vi "Periodic Tasks.vi"(8 "error in":errorcluster) -> ()   [LabVIEW 2017]
doc: "This VI runs in parallel to other tasks. It can contain as many user-defined periodic loops as you need. These can carry out PID or other sorts of timed response."
uses:
  Globals/Global_STOP.vi
  Systems/VisionHW Folder/VisionHW.lvlib
  Systems/Gimbal/Gimbal.lvlib
  _SHARE ALL/RoboRio Share All/Systems Share All/Joystick/Joystick.lvlib
panel:
  in  "Camera Occurance":refnum<k4>
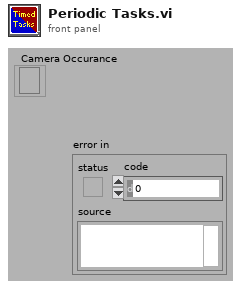
[diagram p1: front panel]
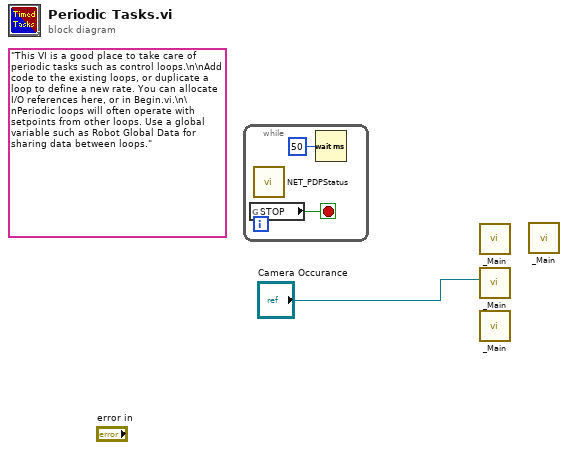
[diagram p0: block diagram]
diagram:
  (unwired) "This VI is a good place to take care of periodic tasks such as control loops.\n\nAdd code to the existing loops, or duplicate a loop to define a new rate. You can allocate I/O references here, or in Begin.vi.\n\nPeriodic loops will often operate with setpoints from other loops. Use a global variable such as Robot Global Data for sharing data between loops."
  n1 = while {
    stop <- w3 stop-if-true
    n2 = global read "Global_STOP.vi" "STOP"() -> (w3:bool)
    n3 = call "NET_PDPStatus.vi"() -> ()  [unwired: 11 in, 1 out]
    n4 = Wait (ms)(milliseconds to wait=u32 50) -> ()  [unwired: 1 out]
  }
  n5 = call "_Main.vi"() -> ()  [unwired: 12 in]
  n6 = call "_Main.vi"("Camera Occurance"="Camera Occurance") -> ()  [unwired: 11 in]
  n7 = call "_Main.vi"() -> ()  [unwired: 12 in]
  n8 = call "_Main.vi"() -> ()  [unwired: 12 in]
